vi "Check ACQ Status_Dual_20230131.vi"(0 "Device Session.lvclass":refnum<class "Device Session.lvclass">, 5 "record count 0":u64, 7 "fetch relative to":T4, 9 "fetch offset":i64, 11 "error in":errorcluster, 12 "record count 1":u64) -> (2 "done":bool, 3 "record status":T2, 4 "Device Session.lvclass 2":refnum<class "Device Session.lvclass">, 6 "fetch backlog":u64[](array[numeric]), 8 "number of outstanding record requests":u32, 10 "records done":u64[](array[numeric]), 13 "overflow occurred":bool, 14 "current record status":T1, 15 "error out":errorcluster)   [LabVIEW 2021, in "Device Session.lvclass"]
doc: "Checks the overall status of the device and reports whether it is operating correctly. This VI checks for system monitor alarms, such as temperature error, power error, FPGA voltage errors, clock PLL lock errors, and channel overload errors.\n\n<B>Input Parameters</B>\n\n<B>device session in</B> is a reference to the Device Session object, which contains a session to each instrument design library used in this sample project. This parameter is obtained from the 'Open Session' VI.\n\n<B>error in</B> describes error conditions that occur before this node runs. This input provides standard 'error in' functionality.\n\n<B>Output Parameters</B>\n\n<B>device session out</B> passes a reference to the session to the next VI.\n\n<B>error out</B> contains error information. This output provides standard 'error out' functionality."
uses:
  Device Session.lvclass
  <instrlib>/_niInstr/Multirecord Acquisition/Interface/v1/Host/Public/Fetch Relative To Enum.ctl
  <instrlib>/_niInstr/Multirecord Acquisition/Interface/v1/Host/Public/Full Record Status.ctl
  <instrlib>/_niInstr/Multirecord Acquisition/Interface/v1/Host/Public/Record State.ctl
  <instrlib>/_niInstr/Multirecord Acquisition/Interface/v1/Host/Public/Record Status.ctl
  Device Session.lvclass/Device Session.ctl
  <instrlib>/_niInstr/Multirecord Acquisition/Interface/v1/Host/niInstr Multirecord Acquisition v1 Host.lvclass
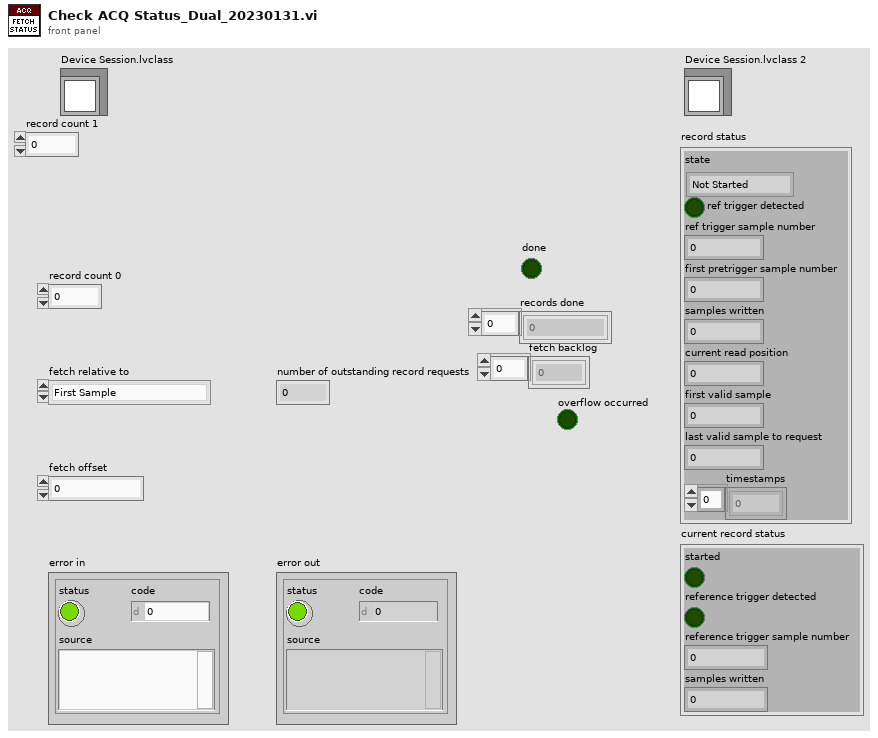
[diagram p1: front panel]
types:
  T1 = typedef "niInstr Multirecord Acquisition v1 Host.lvclass/Record Status.ctl" = cluster{"started":bool, "reference trigger detected":bool, "reference trigger sample number":u64, "samples written":u64}
  T2 = typedef "niInstr Multirecord Acquisition v1 Host.lvclass/Full Record Status.ctl" = cluster{"state":T3, "ref trigger detected":bool, "ref trigger sample number":u64, "first pretrigger sample number":u64, "samples written":u64, "current read position":u64, "first valid sample":u64, "last valid sample to request":u64, "timestamps":u64[]}
  T3 = typedef "niInstr Multirecord Acquisition v1 Host.lvclass/Record State.ctl" = enum16{"Not Started", "Being Acquired", "Completed", "Overwritten"}
  T4 = typedef "niInstr Multirecord Acquisition v1 Host.lvclass/Fetch Relative To Enum.ctl" = enum16{"First Sample", "Reference Trigger Sample", "First Pretrigger Sample", "Most Recent Sample", "Current Read Position"}
  T5 = typedef "Device Session.lvclass/Device Session Object.ctl" = cluster{"fpga reference":T6, "reg bus":refnum<class "niInstr FIFO Register Bus v1 Host.lvclass">, "subsystem map":refnum<class "niInstr Subsystem Map v1 Host.lvclass">, "cal data":refnum<class "niHSAI Cal Data v1 Host.lvclass">, "config":refnum<class "niHSAI Group A Config v1 Host.lvclass">, "acquisition 0":refnum<class "niInstr Multirecord Acquisition v1 Host.lvclass">, "acquisition 1":refnum<class "niInstr Multirecord Acquisition v1 Host.lvclass">, "acquisition 2":refnum<class "niInstr Multirecord Acquisition v1 Host.lvclass">, "acquisition 3":refnum<class "niInstr Multirecord Acquisition v1 Host.lvclass">, "acquisition 4":refnum<class "niInstr Multirecord Acquisition v1 Host.lvclass">, "acquisition 5":refnum<class "niInstr Multirecord Acquisition v1 Host.lvclass">, "acquisition 6":refnum<class "niInstr Multirecord Acquisition v1 Host.lvclass">, "acquisition 7":refnum<class "niInstr Multirecord Acquisition v1 Host.lvclass">, "number of selected acq channels":u8, "selected acq channels":bool[], "number of channels":u32, "configured channels":bool[], "acq configuration":cluster{"number of samples":u64, "number of records":u64, "pretrigger samples":u64}, "actual channel configuration":T7[], "sample clock rate (Hz)":dbl, "scaling coefficients":T11[]}
  T6 = typedef "Device Session.lvclass/FPGA Refnum.ctl" = refnum<k20>
  T7 = typedef "niHSAI Types v1 Host.lvlib/Channel Configuration.ctl" = cluster{"channel":u32, "coupling":T8, "impedance":T9, "bandwidth":T10, "vertical range":dbl, "vertical offset":dbl}
  T8 = typedef "niHSAI Types v1 Host.lvlib/Coupling.ctl" = enum8{"Default", "DC", "AC"}
  T9 = typedef "niHSAI Types v1 Host.lvlib/Impedance.ctl" = enum8{"Default", "1 mega ohm", "50 ohm"}
  T10 = typedef "niHSAI Types v1 Host.lvlib/Bandwidth.ctl" = enum8{"Default", "Full Bandwidth", "Anti-alias Filter", "150 MHz"}
  T11 = typedef "niInstr Multirecord Acquisition v1 Host.lvclass/Scaling Coefficient.ctl" = cluster{"gain":dbl, "offset":dbl}
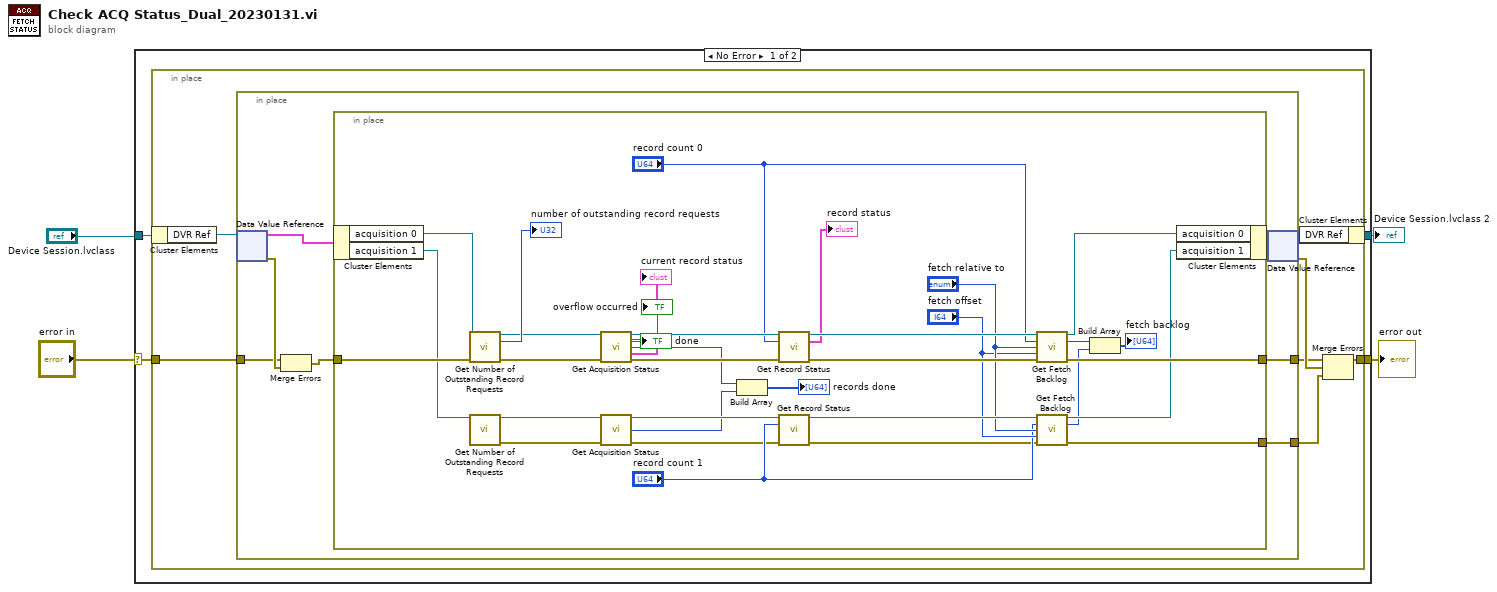
[diagram p0: block diagram]
diagram:
  n1 = case shown="No Error" "error in" {
    selector: "error in" -> [w8 w58]
    tunnel: "Device Session.lvclass" -> [w6 w57]
    tunnel: [w5 w57] -> w1
    tunnel: [w7 w58] -> w3
    frame No Error {
      n2 = in-place {
        in-place-border: w8 -> [w15]
        in-place-border: [w12] -> w7
        n3 = in-place-cluster #1(w6) -> ("DVR Ref"=w11:refnum<data-value>)
        n4 = in-place {
          in-place-border: w15 -> [w19]
          in-place-border: [w22] -> w13
          in-place-border: [w16] -> w9
          n5 = in-place-dvr #2(w11) -> (w18:T5, w20:errorcluster)
          n6 = Merge Errors(w19, w20) -> (w21:errorcluster)
          n7 = in-place {
            in-place-border: [w56] -> w22
            in-place-border: w21 -> [w53]
            in-place-border: [w27] -> w16
            n8 = in-place-cluster #3(w18) -> ("acquisition 0"=w54:refnum<class "niInstr Multirecord Acquisition v1 Host.lvclass">, "acquisition 1"=w38:refnum<class "niInstr Multirecord Acquisition v1 Host.lvclass">)
            n9 = call-dynamic "Get Number of Outstanding Record Requests.vi"("session in"=w54, "error in"=w53) -> ("session out"=w47:refnum<class "niInstr Multirecord Acquisition v1 Host.lvclass">, "number of outstanding record requests"=→"number of outstanding record requests":u32, "error out"=w46:errorcluster)  [unwired: 11 in]
            n10 = call-dynamic "Get Number of Outstanding Record Requests.vi"("session in"=w38) -> ("session out"=w37:refnum<class "niInstr Multirecord Acquisition v1 Host.lvclass">, "error out"=w30:errorcluster)  [unwired: 12 in, 1 out]
            n11 = call-dynamic "Get Acquisition Status.vi"("session in"=w47, "error in"=w46) -> ("overflow occurred"=→"overflow occurred":bool, "session out"=w51:refnum<class "niInstr Multirecord Acquisition v1 Host.lvclass">, "done"=→"done":bool, "records done"=w41:u64, "current record status"=→"current record status":T1, "error out"=w50:errorcluster)  [unwired: 8 in]
            n12 = call-dynamic "Get Acquisition Status.vi"("session in"=w37, "error in"=w30) -> ("session out"=w36:refnum<class "niInstr Multirecord Acquisition v1 Host.lvclass">, "records done"=w25:u64, "error out"=w29:errorcluster)  [unwired: 8 in, 3 out]
            n13 = Build Array(w41, w25) -> (→"records done":u64[])
            n14 = call-dynamic "Get Record Status.vi"("session in"=w51, "record number"="record count 0", "error in"=w50) -> ("session out"=w49:refnum<class "niInstr Multirecord Acquisition v1 Host.lvclass">, "record status"=→"record status":T2, "error out"=w48:errorcluster)  [unwired: 10 in]
            n15 = call-dynamic "Get Record Status.vi"("session in"=w36, "record number"="record count 1", "error in"=w29) -> ("session out"=w35:refnum<class "niInstr Multirecord Acquisition v1 Host.lvclass">, "error out"=w28:errorcluster)  [unwired: 10 in, 1 out]
            n16 = call-dynamic "Get Fetch Backlog.vi"("session in"=w49, "record number"="record count 0", "fetch relative to"="fetch relative to", "fetch offset"="fetch offset", "error in"=w48) -> ("session out"=w55:refnum<class "niInstr Multirecord Acquisition v1 Host.lvclass">, "fetch backlog"=w39:u64, "error out"=w56:errorcluster)  [unwired: 8 in]
            n17 = call-dynamic "Get Fetch Backlog.vi"("session in"=w35, "record number"="record count 1", "fetch relative to"="fetch relative to", "fetch offset"="fetch offset", "error in"=w28) -> ("session out"=w34:refnum<class "niInstr Multirecord Acquisition v1 Host.lvclass">, "fetch backlog"=w23:u64, "error out"=w27:errorcluster)  [unwired: 8 in]
            n18 = Build Array(w39, w23) -> (→"fetch backlog":u64[])
            n19 = in-place-cluster #3("acquisition 0"=w55, "acquisition 1"=w34) -> (w17:T5)
          }
          n20 = in-place-dvr #2(w17) -> (w10:refnum<data-value>, w14:errorcluster)
        }
        n21 = in-place-cluster #1("DVR Ref"=w10) -> (w5:refnum<class "Device Session.lvclass">)
        n22 = Merge Errors(w13, w14, w9) -> (w12:errorcluster)
      }
    }
    frame Error {
    }
  }
  "error out" <- w3
  "Device Session.lvclass 2" <- w1
